vi "Global odometry.vi"() -> ()   [LabVIEW 2023]
uses:
  ctrl defs/ctrl driver input.ctl
  ctrl defs/ctrl swerve module.ctl
  ctrl defs/ctrl XY coord.ctl
  <vilib>/Rock Robotics/WPI/DriverStation/WPI_DriverStationAllianceInfo.ctl
  ctrl defs/ctrl DRIVING FRAME selector.ctl
  ctrl defs/ctrl FRONT FACE selector.ctl
  ctrl defs/ctrl LimeLight target.ctl
  ctrl defs/ctrl swerve speeds.ctl
  ctrl defs/ctrl DRIVER MODE.ctl
  ctrl defs/ctrl pivot select.ctl
  ctrl defs/ctrl PARKING constants.ctl
  ctrl defs/ctrl ROTATION SELECT.ctl
  ctrl defs/ctrl LED PATTERN DEFS.ctl
  ctrl defs/ctrl DRIVER target assist.ctl
panel:
  in  "Tab Control":enum32{"settings", "updates"}(tab)
  out "Driver Assist":T1={"ASSIST?"=FALSE, "LOCKED ON?"=FALSE, "DistanceToTarget (in)"=26.235051697949295, "BRNG (deg)"=-2.0}
  in  "LED PATTERN":T2=enum."COLOR 1 scan COLOR 2"
  in  "DRIVE EFF":dbl=84.886
  in  "DRIVE ROTATION":T3=enum."TWIST axis"
  in  "PARKING":T4={"angle (deg)"=180.0, "%VBus"=0.1} {"%VBus" format="%.4g"; "angle (deg)" format="%_4f"}
  in  "select pivot point":T5
  in  "DRIVER MODE":T6
  in  "SWERVE speeds":T7={"NORMAL"={"DRIVE"=1.0, "STEER"=0.75}, "TURTLE"={"DRIVE"=0.35, "STEER"=0.35}, "TURBO"={"DRIVE"=1.0, "STEER"=1.0}} {"TURBO"."STEER" min=0.02 max=1.0 format="%.3f"; "TURBO"."DRIVE" min=0.02 max=1.0 format="%.3f"; "TURTLE"."STEER" min=0.02 max=1.0 format="%.3f"; "TURTLE"."DRIVE" min=0.02 max=1.0 format="%.3f"; "NORMAL"."STEER" min=0.02 max=1.0 format="%.3f"; "NORMAL"."DRIVE" min=0.02 max=1.0 format="%.3f"}
  in  "Limelight target":T8
  in  "front face":T9
  in  "drive frame":T10
  in  "Alliance":T11
  in  "MAGNETIC Zero for Blue Alliance (deg)":dbl=200.5 format="%#.4f"
  in  "pivot center":T12 {"Y" format="%.4g"; "X" format="%.4g"}
  in  "DRIVER INPUT":T13={"Jx"=0.0, "Jy"=0.0, "Jr "=0.0, "R"=0.0, "theta (deg)"=90.0, "theta (rad)"=1.5707963267948966, "PARK"=FALSE} {"Jr" format="%.4g"; "theta (rad)" format="%_4f"; "R" format="%.4g"; "Jy" format="%.4g"; "theta (deg)" format="%_4f"; "Jx" format="%.4g"}
  out "Continuous Angle":T14
  in  "YRPHfH":T15={"Yaw"=129.52, "Roll"=0.02, "Pitch"=-0.05, "Heading"=270.74, "Fused Heading"=129.25}
  in  "swerve module data":T16[](array[typedef])=[{"descr"="FR", "V"=0.0, "POS"=89.736328125, "target"=0.0, "ABS"=89.82421875, "from pivot to module"={"R"=17.273204450824984, "theta (deg)"=45.0, "theta spin (deg)"=135.0, "theta park (deg)"=0.0}, "coord wrt geom CTR"={"X"=12.214, "Y"=12.214}, "corner wt (lbm)"=37.6}, {"descr"="FL", "V"=0.0, "POS"=271.23046875, "target"=0.0, "ABS"=271.23046875, "from pivot to module"={"R"=17.273204450824984, "theta (deg)"=135.0, "theta spin (deg)"=225.0, "theta park (deg)"=0.0}, "coord wrt geom CTR"={"X"=-12.214, "Y"=12.214}, "corner wt (lbm)"=28.0}, {"descr"="RL", "V"=0.0, "POS"=88.9453125, "target"=0.0, "ABS"=89.033203125, "from pivot to module"={"R"=17.273204450824984, "theta (deg)"=-135.0, "theta spin (deg)"=-45.0, "theta park (deg)"=0.0}, "coord wrt geom CTR"={"X"=-12.214, "Y"=-12.214}, "corner wt (lbm)"=42.6}, {"descr"="RR", "V"=0.0, "POS"=271.7578125, "target"=0.0, "ABS"=271.669921875, "from pivot to module"={"R"=17.273204450824984, "theta (deg)"=-45.0, "theta spin (deg)"=45.0, "theta park (deg)"=0.0}, "coord wrt geom CTR"={"X"=12.214, "Y"=-12.214}, "corner wt (lbm)"=29.8}] {"corner wt (lbm)" format="%#.3f"; "POS" format="%.3g"; "coord wrt geom CTR"."Y" format="%.4g"; "coord wrt geom CTR"."X" format="%.4g"; "from pivot to module"."theta park (deg)" format="%.4g"; "from pivot to module"."theta spin (deg)" format="%.4g"; "from pivot to module"."theta (deg)" format="%.4g"; "from pivot to module"."R" format="%.4g"; "ABS" format="%.3g"; "target" format="%.3g"; "V" format="%.3g"}
  in  "RUN ARMS":T17={"LEFT ARM"={"VBus%"=0.0, "LOCK?"=TRUE, "LOCKED"=FALSE}, "RIGHT ARM"={"VBus%"=0.0, "LOCK?"=TRUE, "LOCKED"=FALSE}} {"RIGHT ARM"."VBus%" min=-1.0 max=1.0 step=0.005 format="%#.5f"; "LEFT ARM"."VBus%" min=-1.0 max=1.0 step=0.005 format="%#.5f"}
  # "NOTE on driving speeds:\n     NEO motor free speed = 5676 rpm\n     drive gearing = 6.75\n     max wheel rotation = 5676 / 6.75 = 841 rpm\n     4\" wheel diam = 4*pi = 12.5664 in/rev travel\n\ntheoretical 100% speed = (841 rpm)*1/60*(4in*pi)\n     =  176.14 in/s  =  14.67 ft/s\n\n- check SWERVE SPEEDS as joystick values may max out to value\n\ndistance (ft) = (%eff/100)14.67*(%th/100)*(time(ms) / 1000)\n\ntime (ms) = (10^7)*distance (ft) / (14.67*%th*%eff)"
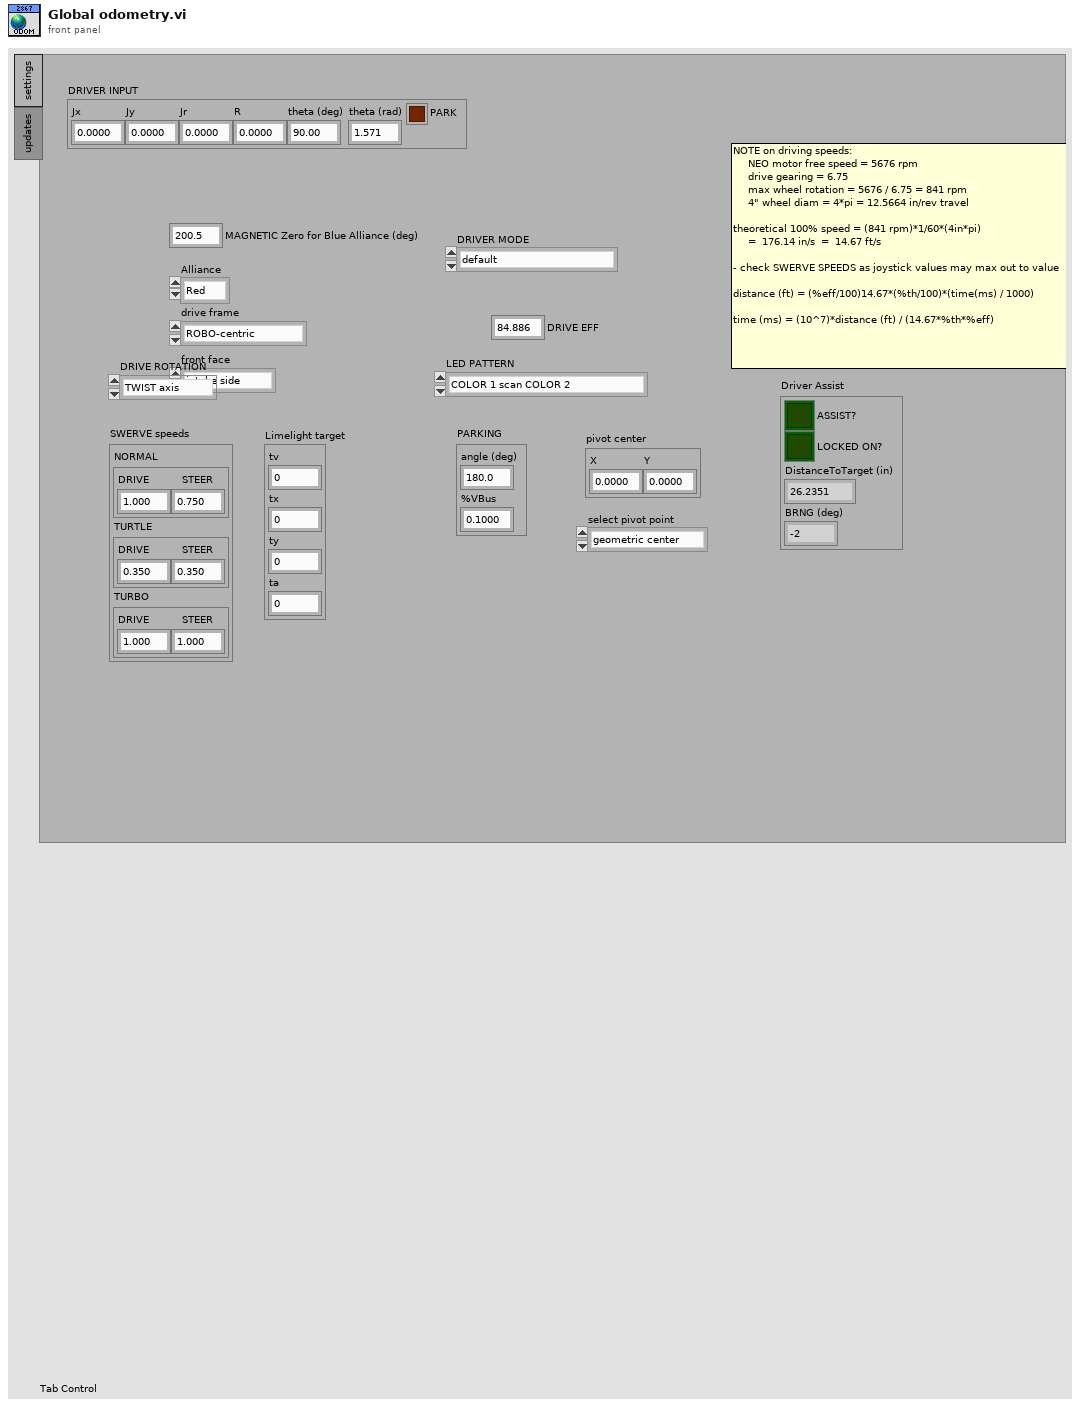
[diagram p1: front panel]
types:
  T1 = typedef "ctrl DRIVER target assist.ctl" = cluster{"ASSIST?":bool, "LOCKED ON?":bool, "DistanceToTarget (in)":dbl, "BRNG (deg)":dbl}
  T2 = typedef "ctrl LED PATTERN DEFS.ctl" = enum16{"default", "RED, SOLID", "RED, BUMPER", "RED, BLINK", "RED, WAVE", "RED, SCAN", "RED, PULSE", "BLUE, SOLID", "BLUE, BUMPER", "BLUE, BLINK", "BLUE, WAVE", "BLUE, SCAN", "BLUE, PULSE", "GREEN, SOLID", "GREEN, BUMPER", "GREEN, BLINK", "GREEN, WAVE", "GREEN, SCAN", "GREEN, PULSE", "WHITE, WAVE", "WHITE, PULSE", "COLOR 1 scan white", "COLOR 1 scan COLOR 2", "COLOR 1 bumper white", "COLOR 1 bumper COLOR 2", "PINK, SOLID", "PINK, BLINK", "VIOLET, SOLID", "VIOLET, BLINK", "ORANGE, SOLID", "ORANGE, BLINK", "YELLOW, SOLID", "YELLOW, BLINK", "FUSCIA, SOLID", "FUSCIA, BLINK", "AQUA, SOLID", "AQUA, BLINK", "AQUA, BUMPER", "AQUA, SCAN", "FUSCIA, BUMPER", "FUSCIA, SCAN", "ORANGE, BUMPER", "ORANGE, SCAN", "VIOLET, BUMPER", "VIOLET, SCAN", "YELLOW, BUMPER", "YELLOW, SCAN", "PINK, BUMPER", "PINK, SCAN", "CROSSING, RED & BLUE", "CROSSING, COLORS 1&2", "TEST", "RAINBOW", "RED, EXPAND", "BLUE, EXPAND", "GREEN, EXPAND", "RED, EX-CON", "BLUE, EX-CON", "GREEN, EX-CON", "EMERGENCY STOP", "LOW BATTERY"}
  T3 = typedef "ctrl ROTATION SELECT.ctl" = enum16{"POV hat ", "TWIST axis"}
  T4 = typedef "ctrl PARKING constants.ctl" = cluster{"angle (deg)":dbl, "%VBus":dbl}
  T5 = typedef "ctrl pivot select.ctl" = enum16{"geometric center", "CG", "FL", "FR", "RR", "RL", "other"}
  T6 = typedef "ctrl DRIVER MODE.ctl" = enum16{"default", "TURTLE", "TURBO"}
  T7 = typedef "ctrl swerve speeds.ctl" = cluster{"NORMAL":cluster{"DRIVE":dbl, "STEER":dbl}, "TURTLE":cluster{"DRIVE":dbl, "STEER":dbl}, "TURBO":cluster{"DRIVE":dbl, "STEER":dbl}}
  T8 = typedef "ctrl LimeLight target.ctl" = cluster{"tv":u8, "tx":dbl, "ty":dbl, "ta":dbl}
  T9 = typedef "ctrl FRONT FACE selector.ctl" = enum16{"intake side", "shooter side"}
  T10 = typedef "ctrl DRIVING FRAME selector.ctl" = enum16{"ROBO-centric", "FLD-centric"}
  T11 = typedef "WPI_DriverStationAllianceInfo.ctl" = enum16{"Red", "Blue", "Invalid"}
  T12 = typedef "ctrl XY coord.ctl" = cluster{"X":dbl, "Y":dbl}
  T13 = typedef "ctrl driver input.ctl" = cluster{"Jx":dbl, "Jy":dbl, "Jr ":dbl, "R":dbl, "theta (deg)":dbl, "theta (rad)":dbl, "PARK":bool}
  T14 = cluster{"Rollover":dbl, "Yaw":dbl, "Cont Yaw":dbl}
  T15 = cluster{"Yaw":dbl, "Roll":dbl, "Pitch":dbl, "Heading":dbl, "Fused Heading":dbl}
  T16 = typedef "ctrl swerve module.ctl" = cluster{"descr":string, "V":dbl, "POS":dbl, "target":dbl, "ABS":dbl, "from pivot to module":cluster{"R":dbl, "theta (deg)":dbl, "theta spin (deg)":dbl, "theta park (deg)":dbl}, "coord wrt geom CTR":cluster{"X":dbl, "Y":dbl}, "corner wt (lbm)":dbl}
  T17 = cluster{"LEFT ARM":cluster{"VBus%":dbl, "LOCK?":bool, "LOCKED":bool}, "RIGHT ARM":cluster{"VBus%":dbl, "LOCK?":bool, "LOCKED":bool}}
diagram:
